vi "Get Item Tag.vi"(8 "error in (no error)":errorcluster, 9 "Active Cell:Active Column Number":i32, 10 "Active Item:Tag":string, 11 "reference":refnum<vi>) -> (0 "error out":errorcluster, 2 "Active Cell:String":string, 3 "reference out":refnum<vi>)   [LabVIEW 2019, in "Tree Control.lvlib"]
doc: "Get Item Tag from Tree Control."
uses:
  Tree Control.lvlib
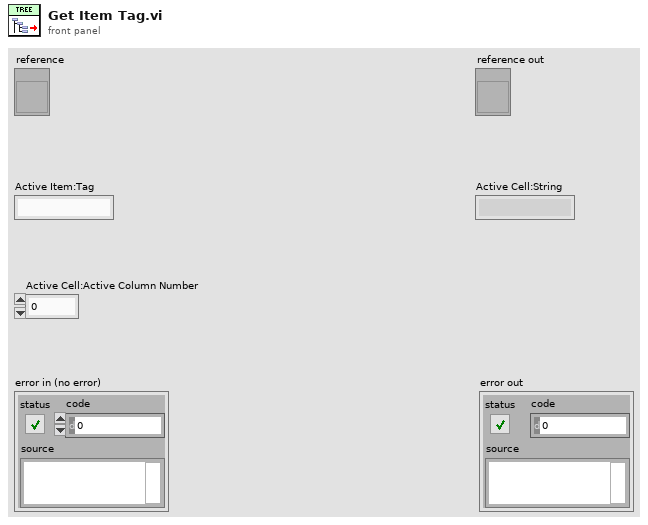
[diagram p1: front panel]
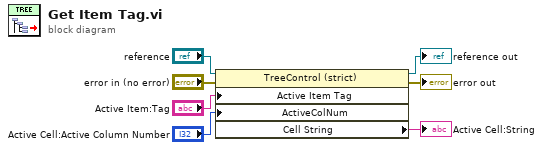
[diagram p0: block diagram]
diagram:
  n1 = property on="Property Node" class="TreeControl (strict)"(reference="reference", error in="error in (no error)", "Active Item Tag"="Active Item:Tag", "ActiveColNum"="Active Cell:Active Column Number") -> (reference out=→"reference out":refnum<vi>, error out=→"error out":errorcluster, "Cell String"=→"Active Cell:String":string)
